vi "Plugin - Current Time.vi"() -> ()   [LabVIEW 2014]
doc: "Subpanel Plugin VI that displays the current time."
panel:
  out "Current Time":string
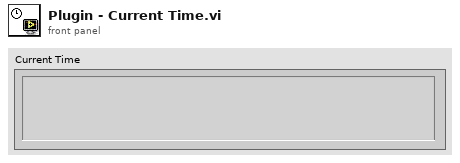
[diagram p1: front panel]
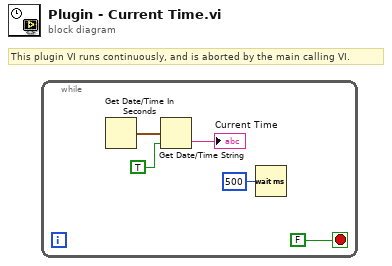
[diagram p0: block diagram]
diagram:
  # "This plugin VI runs continuously, and is aborted by the main calling VI."
  n1 = while {
    stop <- FALSE stop-if-true
    n2 = Get Date/Time In Seconds() -> (seconds since 1Jan1904=w5:timestamp)
    n3 = Get Date/Time String(seconds (now)=w5, want seconds? (F)=TRUE) -> (time string=→"Current Time":string)  [unwired: 1 in, 1 out]
    n4 = Wait (ms)(milliseconds to wait=u32 500) -> ()  [unwired: 1 out]
  }
